vi "Compare Clusters.vi"(1 "PS4 Controller":T1 {"R2" scale=-32768.0..32767.0; "L2" scale=-32768.0..32767.0}) -> (0 "Checkbox":bool)   [LabVIEW 2021]
uses:
  <vilib>/MakerHub/PS4-Controller/Private/Type Defs/Indicators/Controller.ctl
  <vilib>/MakerHub/PS4-Controller/Private/Type Defs/Indicators/Square.ctl
  <vilib>/MakerHub/PS4-Controller/Private/Type Defs/Indicators/X.ctl
  <vilib>/MakerHub/PS4-Controller/Private/Type Defs/Indicators/Circle.ctl
  <vilib>/MakerHub/PS4-Controller/Private/Type Defs/Indicators/Triangle.ctl
  <vilib>/MakerHub/PS4-Controller/Private/Type Defs/Indicators/L1.ctl
  <vilib>/MakerHub/PS4-Controller/Private/Type Defs/Indicators/R1.ctl
  <vilib>/MakerHub/PS4-Controller/Private/Type Defs/Indicators/Share.ctl
  <vilib>/MakerHub/PS4-Controller/Private/Type Defs/Indicators/Options.ctl
  <vilib>/MakerHub/PS4-Controller/Private/Type Defs/Indicators/PS.ctl
  <vilib>/MakerHub/PS4-Controller/Private/Type Defs/Indicators/Pad_Button.ctl
  <vilib>/MakerHub/PS4-Controller/Private/Type Defs/Indicators/Dpad.ctl
  <vilib>/MakerHub/PS4-Controller/Private/Type Defs/Indicators/Slider.ctl
  <vilib>/MakerHub/PS4-Controller/LMH-PS4.lvlib
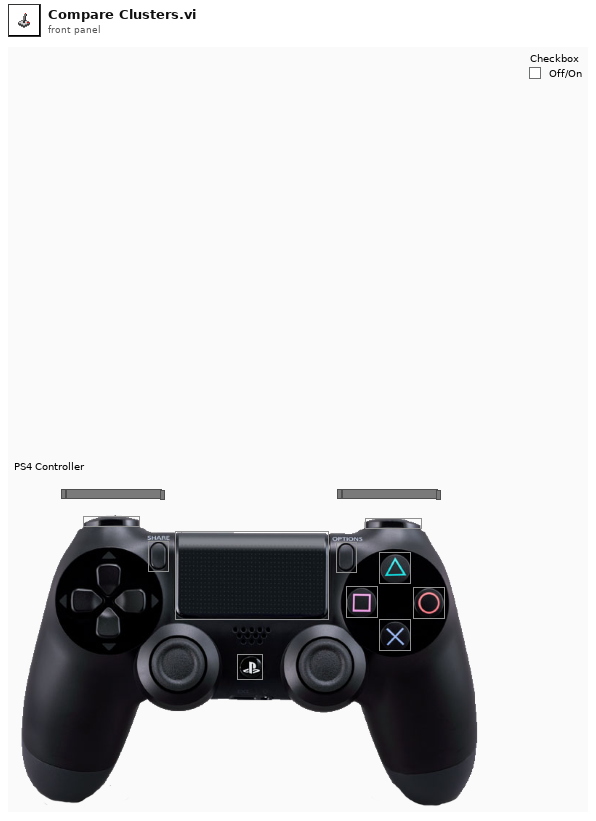
[diagram p1: front panel]
types:
  T1 = typedef "LMH-PS4.lvlib/Controller.ctl" = cluster{"Square Button":T2, "X Button":T3, "Circle Button":T4, "Triangle Button":T5, "L1":T6, "R1":T7, "Share Button":T8, "Options Button":T9, "PS Button":T10, "Pad Button":T11, "D-Pad":T12, "L2":T13, "R2":T13, "Thumbstick_Left":cluster{i32[], i32[]}, "Thumbstick_Right":cluster{i32[], i32[]}}
  T2 = typedef "LMH-PS4.lvlib/Square.ctl" = bool
  T3 = typedef "LMH-PS4.lvlib/X.ctl" = bool
  T4 = typedef "LMH-PS4.lvlib/Circle.ctl" = bool
  T5 = typedef "LMH-PS4.lvlib/Triangle.ctl" = bool
  T6 = typedef "LMH-PS4.lvlib/L1.ctl" = bool
  T7 = typedef "LMH-PS4.lvlib/R1.ctl" = bool
  T8 = typedef "LMH-PS4.lvlib/Share.ctl" = bool
  T9 = typedef "LMH-PS4.lvlib/Options.ctl" = bool
  T10 = typedef "LMH-PS4.lvlib/PS.ctl" = bool
  T11 = typedef "LMH-PS4.lvlib/Pad_Button.ctl" = bool
  T12 = typedef "LMH-PS4.lvlib/Dpad.ctl" = u16
  T13 = typedef "LMH-PS4.lvlib/Slider.ctl" = i32
  T14 = cluster{"Square Button":T2, "Circle Button":T4, "X Button":T3, "L2":T13, "R2":T13}
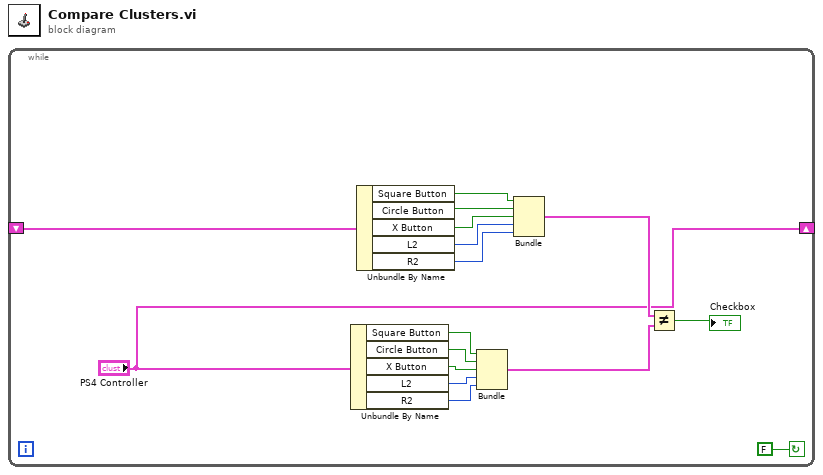
[diagram p0: block diagram]
diagram:
  n1 = while {
    shift-right: ["PS4 Controller"] -> _
    shift-left: _ -> [w2]
    stop <- FALSE continue-if-true
    n2 = Unbundle By Name("PS4 Controller") -> ("Square Button"=w11:T2, "Circle Button"=w12:T4, "X Button"=w13:T3, "L2"=w14:T13, "R2"=w15:T13)
    n3 = Unbundle By Name(w2) -> ("Square Button"=w6:T2, "Circle Button"=w7:T4, "X Button"=w8:T3, "L2"=w9:T13, "R2"=w10:T13)
    n4 = Bundle("Square Button"=w11, "Circle Button"=w12, "X Button"=w13, "L2"=w14, "R2"=w15) -> (w16:T14)  [unwired: 1 in]
    n5 = Bundle("Square Button"=w6, "Circle Button"=w7, "X Button"=w8, "L2"=w9, "R2"=w10) -> (w3:T14)  [unwired: 1 in]
    n6 = Not Equal?(x=w3, y=w16) -> (x != y?=→"Checkbox":bool)
  }
